vi "Physical Constants to XML.vi"() -> (0 "XML Data":string)   [LabVIEW 2013]
uses:
  Types/Physical Constants.ctl
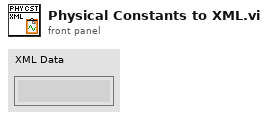
[diagram p1: front panel]
types:
  T1 = typedef "Physical Constants.ctl" = cluster{"Maximum Input Voltage":dbl, "Maximum Output Voltage":dbl, "Minimum Input Voltage":dbl, "Minimum Output Voltage":dbl, "X Maximum Extension":dbl, "X Minimum Extension":dbl, "X Piezo Response":dbl, "Y Maximum Extension":dbl, "Y Minimum Extension":dbl, "Y Piezo Response":dbl, "Z Maximum Extension":dbl, "Z Minimum Extension":dbl, "Z Piezo Response":dbl, "Version":string}
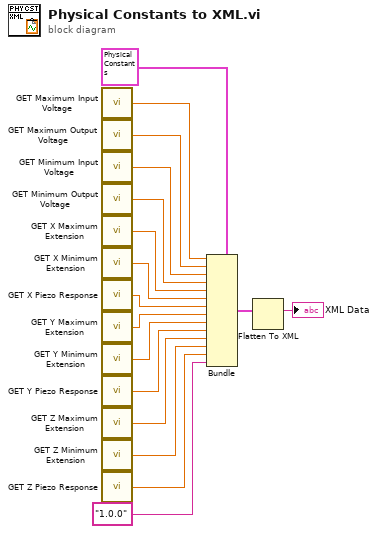
[diagram p0: block diagram]
diagram:
  n1 = call "GET Maximum Input Voltage.vi"() -> ("Maximum Input Voltage"=w8:dbl)
  n2 = call "GET Maximum Output Voltage.vi"() -> ("Maximum Output Voltage"=w9:dbl)
  n3 = call "GET Minimum Input Voltage.vi"() -> ("Minimum Input Voltage"=w10:dbl)
  n4 = call "GET Minimum Output Voltage.vi"() -> ("Minimum Output Voltage"=w11:dbl)
  n5 = call "GET X Maximum Extension.vi"() -> ("X Maximum Extension"=w12:dbl)
  n6 = call "GET X Minimum Extension.vi"() -> ("X Minimum Extension"=w13:dbl)
  n7 = call "GET X Piezo Response.vi"() -> ("X Piezo Response"=w15:dbl)
  n8 = call "GET Y Maximum Extension.vi"() -> ("Y Maximum Extension"=w14:dbl)
  n9 = call "GET Y Minimum Extension.vi"() -> ("Y Minimum Extension"=w7:dbl)
  n10 = call "GET Y Piezo Response.vi"() -> ("Y Piezo Response"=w6:dbl)
  n11 = call "GET Z Maximum Extension.vi"() -> ("Z Maximum Extension"=w5:dbl)
  n12 = call "GET Z Minimum Extension.vi"() -> ("Z Minimum Extension"=w4:dbl)
  n13 = call "GET Z Piezo Response.vi"() -> ("Z Piezo Response"=w3:dbl)
  n14 = Bundle(cluster=T1 {"Maximum Input Voltage"=0.0, "Maximum Output Voltage"=0.0, "Minimum Input Voltage"=0.0, "Minimum Output Voltage"=0.0, "X Maximum Extension"=0.0, "X Minimum Extension"=0.0, "X Piezo Response"=0.0, "Y Maximum Extension"=0.0, "Y Minimum Extension"=0.0, "Y Piezo Response"=0.0, "Z Maximum Extension"=0.0, "Z Minimum Extension"=0.0, "Z Piezo Response"=0.0, "Version"=""} ("Physical Constants"), "Maximum Input Voltage"=w8, "Maximum Output Voltage"=w9, "Minimum Input Voltage"=w10, "Minimum Output Voltage"=w11, "X Maximum Extension"=w12, "X Minimum Extension"=w13, "X Piezo Response"=w15, "Y Maximum Extension"=w14, "Y Minimum Extension"=w7, "Y Piezo Response"=w6, "Z Maximum Extension"=w5, "Z Minimum Extension"=w4, "Z Piezo Response"=w3, "Version"="1.0.0") -> (w17:T1)
  n15 = Flatten To XML(anything=w17) -> (xml string=→"XML Data":string)
